vi "decode fixed32.vi"(10 "read index in":i32, 11 "byte array in":u8[](array[numeric]) format="%.0b") -> (1 "u32":u32, 2 "read index out":i32)   [LabVIEW 2013, in "protocol buffers encoder.lvlib"]
uses:
  protocol buffers encoder.lvlib
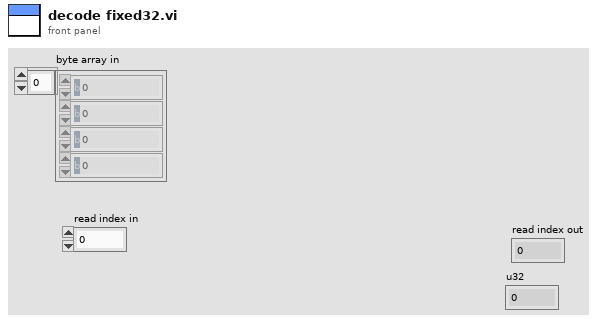
[diagram p1: front panel]
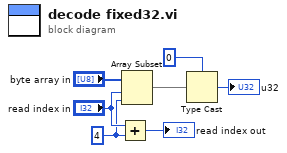
[diagram p0: block diagram]
diagram:
  w4 = 4 ("index")
  n1 = Add(x="read index in", y=w4) -> (x+y=→"read index out":i32)
  n2 = Array Subset(array="byte array in", index="read index in", length=w4) -> (w2:u8[])
  n3 = Type Cast(type=u32 0, x=w2) -> (*(type *) &x=→"u32":u32)
